vi "getPositionABS.vi"(3 "Device":refnum<k24>) -> (1 "GetPOS":dbl)   [LabVIEW 2014]
doc: "Returns the <B>absolute position value</B> of motor.\n\n\nAndré Romero - 2017\nandretec@ifsc.usp.br"
uses:
  C:/UserLabs/Andre/kinesis-lab14-32bits/kinesis-teste/Kinesis/Thorlabs.MotionControl.TCube.DCServoCLI.dll
  Kinesis/Thorlabs.MotionControl.TCube.DCServoCLI.dll
panel:
  out "GetPositionCounter":i32
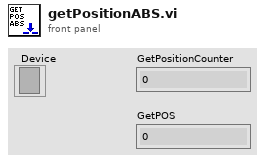
[diagram p1: front panel]
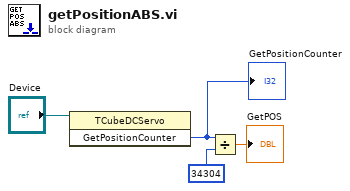
[diagram p0: block diagram]
diagram:
  n1 = invoke class="TCubeDCServo" method="GetPositionCounter"(reference="Device") -> ("GetPositionCounter"=w1:i32)  [unwired: 2 in, 2 out]
  "GetPositionCounter" <- w1
  n2 = Divide(x=w1, y=34304) -> (x/y=→"GetPOS":dbl)
